vi "dump.vi"(8 "error in (no error)":errorcluster, 10 "indent":T1, 11 "Dimension in":refnum<class "Dimension.lvclass">) -> (0 "error out":errorcluster, 2 "mlir":string, 3 "Dimension out":refnum<class "Dimension.lvclass">)   [LabVIEW 2020, in "mlir.lvlib" / "Dimension.lvclass"]
uses:
  Dimension.lvclass
  Node/indent.ctl
  mlir.lvlib
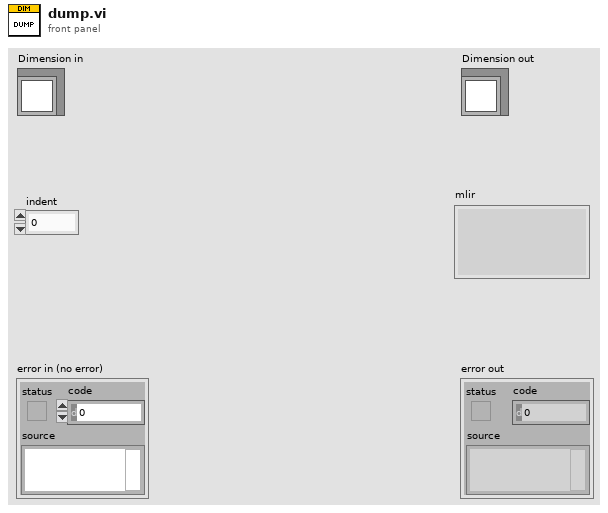
[diagram p1: front panel]
types:
  T1 = typedef "mlir.lvlib/indent.ctl" = u32
  T2 = typedef "mlir.lvlib/Dimension.lvclass/value.ctl" = u32
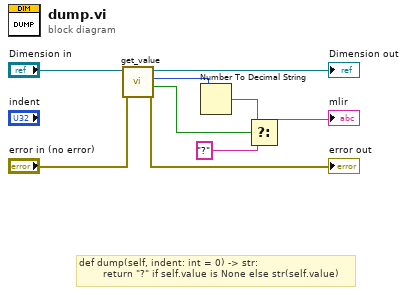
[diagram p0: block diagram]
diagram:
  # "def dump(self, indent: int = 0) -> str:\n        return \"?\" if self.value is None else str(self.value)"
  n1 = call-dynamic "get_value.vi"("error in (no error)"="error in (no error)", "Dimension in"="Dimension in") -> ("error out"=→"error out":errorcluster, "is_set?"=w8:bool, "value"=w6:T2, "Dimension out"=→"Dimension out":refnum<class "Dimension.lvclass">)  [unwired: 6 in]
  n2 = Number To Decimal String(number=w6) -> (decimal integer string=w5:string)  [unwired: 1 in]
  n3 = Select(t=w5, s=w8, f="?") -> (s? t:f=→"mlir":string)
